vi "Stop.vi"(8 "error in (no error)":errorcluster, 11 "L2Enet_RW_CORE in":refnum<class "L2ENET_RW_CORE.lvclass">) -> (0 "error out":errorcluster, 3 "L2Enet_RW_CORE out":refnum<class "L2ENET_RW_CORE.lvclass">)   [LabVIEW 2021, in "L2ENET_RW_CORE.lvclass"]
uses:
  L2ENET_RW_CORE.lvclass
  L2ENET_RW_CORE.lvclass/L2ENET_RW_CORE.ctl
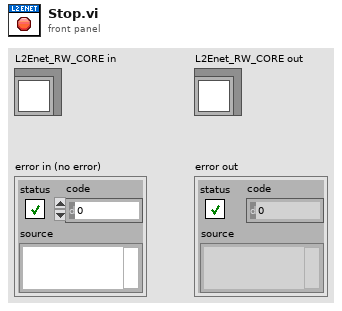
[diagram p1: front panel]
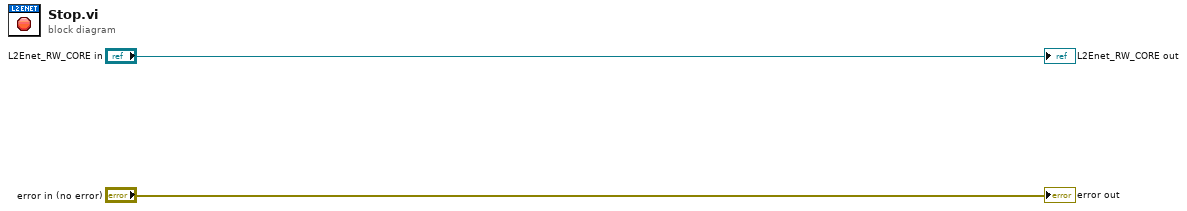
[diagram p0: block diagram]
diagram:
  "error out" <- "error in (no error)"
  "L2Enet_RW_CORE out" <- "L2Enet_RW_CORE in"
